vi "Assign Pixel to Wing Sector (Host).vi"(6 "Pixel Intensity In":u8, 7 "Right Wing?":bool, 8 "Sector Parameters":T1, 9 "Pixel Y":u16, 10 "Pixel X":u16) -> (0 "Pixel Y Out":u16, 1 "Pixel Intensity Out":u8, 2 "sector #":u8, 3 "output valid":bool, 4 "Pixel X Out":u16)   [LabVIEW 2013]
uses:
  FPGA/Sector/Accumulate/Sector Parameter Cluster.ctl
  <vilib>/rvi/FXPMathLib/FxpRectToPolar/subVIs/nifxpmath_RectToPolar_SimConfig.ctl
  <vilib>/rvi/FXPMathLib/FxpDiv/subVIs/nifxpmath_Div_SimConfig.ctl
  <vilib>/rvi/FXPMathLib/FxpRectToPolar/simVIs/DllFxpRectToPolarTemp_sub.vi
  <vilib>/rvi/FXPMathLib/FxpDiv/simVIs/DllFxpDivTemp_sub.vi
  <vilib>/rvi/FXPMathLib/FxpSub/XNode/nifxpmath_Sub.xnode
  <vilib>/rvi/FXPMathLib/FxpRectToPolar/XNode/nifxpmath_RectToPolar.xnode
  <vilib>/rvi/FXPMathLib/FxpAdd/XNode/nifxpmath_Add.xnode
  <vilib>/rvi/FXPMathLib/FxpDiv/XNode/nifxpmath_Div.xnode
  <vilib>/rvi/FXPMathLib/sim/FxpSim.dll
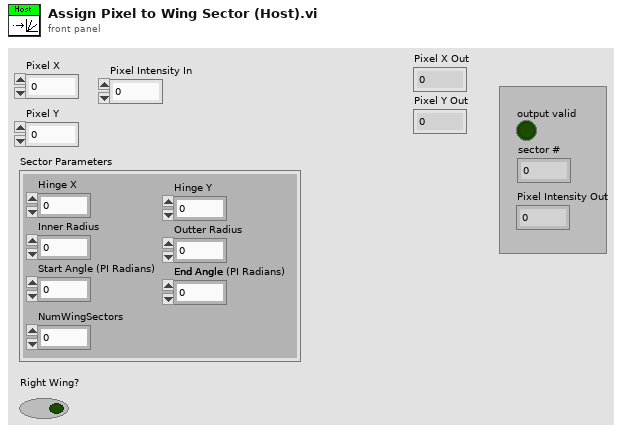
[diagram p1: front panel]
types:
  T1 = typedef "Sector Parameter Cluster.ctl" = cluster{"Start Angle":fxp<+/-,17,2>, "End Angle":fxp<+,17,3>, "Inner Radius":u16, "Outter Radius":u16, "Hinge X":u16, "Hinge Y":u16, "NumWingSectors":u8}
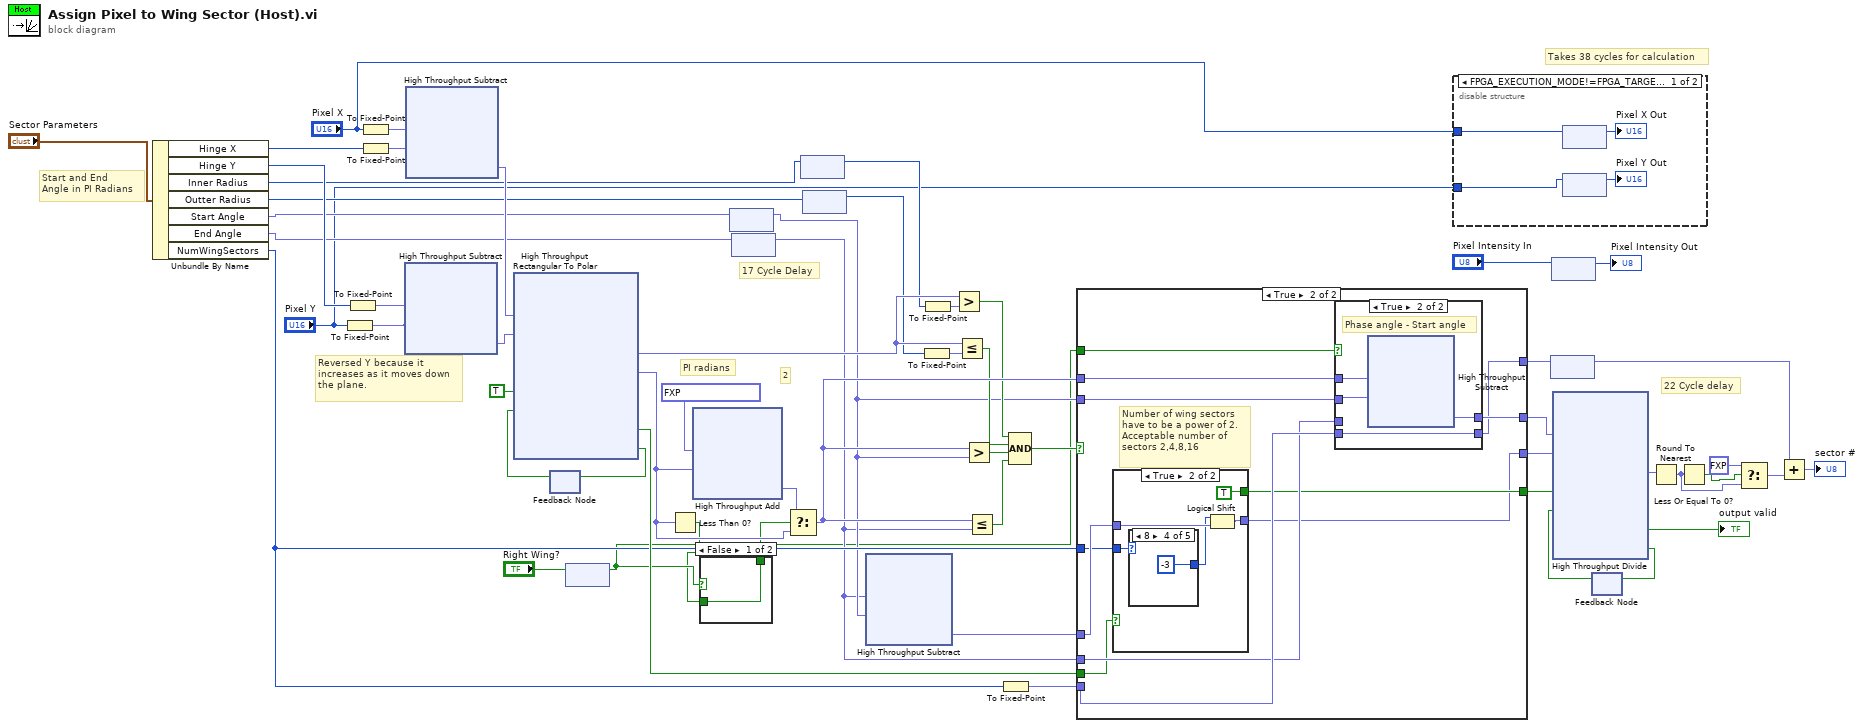
[diagram p0: block diagram]
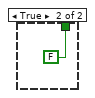
[diagram p2: hidden frame]
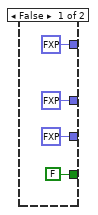
[diagram p4: hidden frame]
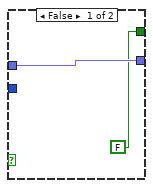
[diagram p5: hidden frame]
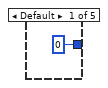
[diagram p6: hidden frame]
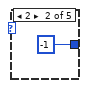
[diagram p7: hidden frame]
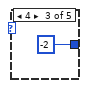
[diagram p8: hidden frame]
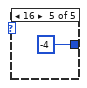
[diagram p9: hidden frame]
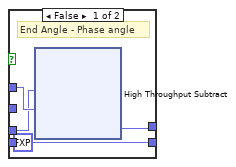
[diagram p10: hidden frame]
diagram:
  # "Takes 38 cycles for calculation"
  # "17 Cycle Delay"
  # "Reversed Y because it\nincreases as it moves down\nthe plane."
  # "PI radians"
  # "22 Cycle delay"
  # "Start and End\nAngle in PI Radians"
  # "2"
  n1 = Unbundle By Name("Sector Parameters") -> ("Hinge X"=w23:u16, "Hinge Y"=w43:u16, "Inner Radius"=w20:u16, "Outter Radius"=w18:u16, "Start Angle"=w16:fxp<+/-,17,2>, "End Angle"=w14:fxp<+,17,3>, "NumWingSectors"=w26:u8)
  n2 = To Fixed-Point(number="Pixel Y") -> (fixed-point=w31:fxp<+,11,11>)  [unwired: 1 in]
  n3 = To Fixed-Point(number=w43) -> (fixed-point=w32:fxp<+,11,11>)  [unwired: 1 in]
  n4 = To Fixed-Point(number="Pixel X") -> (fixed-point=w30:fxp<+,11,11>)  [unwired: 1 in]
  n5 = To Fixed-Point(number=w23) -> (fixed-point=w29:fxp<+,11,11>)  [unwired: 1 in]
  n6 = xnode "High Throughput Subtract"("x"=w32, "y"=w31) -> ("x-y"=w41:fxp<+/-,12,12>)
  n7 = xnode "High Throughput Subtract"("x"=w30, "y"=w29) -> ("x-y"=w40:fxp<+/-,12,12>)
  n8 = feedback #1() -> (w48:bool)  [unwired: 1 in]
  n9 = xnode "High Throughput Rectangular To Polar"("x"=w40, "y"=w41, "input valid"=TRUE, "ready for output (T)"=w48) -> ("magnitude"=w57:fxp<+,12,12>, "phase (pi)"=w54:fxp<+/-,16,2>, "output valid"=w27:bool, "ready for input"=w49:bool)
  n10 = feedback-in #1(w49) -> ()
  n11 = feedback #2() -> (w6:bool)  [unwired: 1 in]
  n12 = feedback-in #2("Right Wing?") -> ()
  n13 = Less Than 0?(x=w54) -> (x < 0?=w5:bool)
  n14 = xnode ("High Throughput Add")("x"=fxp<+/-,16,2> 1.99993896484375 ("y"), "y"=w54) -> ("x+y"=w53:fxp<+/-,17,3>)
  n15 = case shown="False" w6 {
    tunnel: [w59 FALSE ("s")] -> w4
    tunnel: w5 -> [w59 _]
    frame False {
    }
    frame True {
    }
  }
  n16 = feedback #3() -> (w15:fxp<+/-,17,2>)  [unwired: 1 in]
  n17 = feedback-in #3(w16) -> ()
  n18 = feedback #4() -> (w13:fxp<+,17,3>)  [unwired: 1 in]
  n19 = feedback-in #4(w14) -> ()
  n20 = Select(t=w53, s=w4, f=w54) -> (s? t:f=w51:fxp<+/-,17,3>)
  n21 = feedback #5() -> (w19:u16)  [unwired: 1 in]
  n22 = feedback-in #5(w20) -> ()
  n23 = feedback #6() -> (w17:u16)  [unwired: 1 in]
  n24 = feedback-in #6(w18) -> ()
  n25 = xnode ("High Throughput Subtract")("x"=w13, "y"=w15) -> ("x-y"=w28:fxp<+/-,17,6>)
  n26 = To Fixed-Point(number=w17) -> (fixed-point=w56:fxp<+,16,16>)  [unwired: 1 in]
  n27 = To Fixed-Point(number=w19) -> (fixed-point=w58:fxp<+,16,16>)  [unwired: 1 in]
  n28 = Greater?(x=w57, y=w58) -> (0:w47:bool)
  n29 = Less Or Equal?(x=w57, y=w56) -> (x <= y?=w46:bool)
  n30 = Greater?(x=w51, y=w15) -> (0:w45:bool)
  n31 = Less Or Equal?(x=w51, y=w13) -> (x <= y?=w44:bool)
  n32 = To Fixed-Point(number=w26) -> (fixed-point=w42:fxp<+,8,8>)  [unwired: 1 in]
  n33 = Compound Arithmetic op=AND(w47, w46, w45, w44) -> (w55:bool)
  n34 = case shown="True" w55 {
    tunnel: w51 -> [_ w76]
    tunnel: w15 -> [_ w75]
    tunnel: [fxp<+/-,17,6> 0.0 ("x-y") w66] -> w36
    tunnel: w13 -> [_ w73]
    tunnel: w42 -> [_ w74]
    tunnel: [fxp<+/-,19,5> 0.0 ("x-y") w72] -> w37
    tunnel: [FALSE ("output valid") w67] -> w35
    tunnel: [fxp<+,8,8> 0.0 w71] -> w33
    tunnel: w28 -> [_ w70]
    tunnel: w27 -> [_ w69]
    tunnel: w26 -> [_ w68]
    tunnel: w6 -> [_ w65]
    frame False {
    }
    frame True {
      # "Number of wing sectors\nhave to be a power of 2.\nAcceptable number of\nsectors 2,4,8,16"
      n35 = case shown="True" w69 {
        tunnel: w68 -> [_ w83]
        tunnel: w70 -> [w78 w82]
        tunnel: [w78 w80] -> w66
        tunnel: [FALSE ("output valid") TRUE ("output valid")] -> w67
        frame False {
        }
        frame True {
          n36 = case shown="8" w83 {
            tunnel: [i16 0 ("y") i16 -1 ("y") i16 -2 ("y") i16 -3 ("y") i16 -4 ("y")] -> w81
            frame Default {
            }
            frame 2 {
            }
            frame 4 {
            }
            frame 8 {
            }
            frame 16 {
            }
          }
          n37 = Logical Shift(y=w81, x=w82) -> (x << y=w80:fxp<+/-,17,6>)
        }
      }
      n38 = case shown="True" w65 {
        tunnel: w76 -> [w91 w96]
        tunnel: w75 -> [_ w95]
        tunnel: [w92 w94] -> w72
        tunnel: w74 -> [_ w93]
        tunnel: [fxp<+,8,8> 0.0 w93] -> w71
        tunnel: w73 -> [w90 _]
        frame False {
          # "End Angle - Phase angle"
          n39 = xnode "High Throughput Subtract"("x"=w90, "y"=w91) -> ("x-y"=w92:fxp<+/-,19,5>)
        }
        frame True {
          # "Phase angle - Start angle"
          n40 = xnode ("High Throughput Subtract")("x"=w96, "y"=w95) -> ("x-y"=w94:fxp<+/-,19,4>)
        }
      }
    }
  }
  n41 = disable-structure shown="FPGA_EXECUTION_MODE!=FPGA_TARGET" {
    disable-tunnel: "Pixel X" -> [w100 _]
    disable-tunnel: "Pixel Y" -> [w99 _]
    frame condition #0 (active) {
      n42 = feedback #7() -> (→"Pixel X Out":u16)  [unwired: 1 in]
      n43 = feedback-in #7(w100) -> ()
      n44 = feedback #8() -> (→"Pixel Y Out":u16)  [unwired: 1 in]
      n45 = feedback-in #8(w99) -> ()
    }
    frame condition #1 {
    }
  }
  n46 = feedback #9() -> (w10:fxp<+,8,8>)  [unwired: 1 in]
  n47 = feedback-in #9(w33) -> ()
  n48 = feedback #10() -> (→"Pixel Intensity Out":u8)  [unwired: 1 in]
  n49 = feedback-in #10("Pixel Intensity In") -> ()
  n50 = feedback #11() -> (w34:bool)  [unwired: 1 in]
  n51 = xnode "High Throughput Divide"("x"=w37, "y"=w36, "input valid"=w35, "ready for output (T)"=w34) -> ("x/y"=w3:fxp<+/-,20,16>, "output valid"=→"output valid":bool, "ready for input"=w39:bool)
  n52 = feedback-in #11(w39) -> ()
  n53 = Round To Nearest(number=w3) -> (nearest integer value=w1:fxp<+/-,17,17>)
  n54 = Less Or Equal To 0?(x=w1) -> (x <= 0?=w2:bool)
  n55 = Select(t=fxp<+/-,17,17> 1.0, s=w2, f=w1) -> (s? t:f=w12:fxp<+/-,17,17>)
  n56 = Add(x=w10, y=w12) -> (x+y=→"sector #":fxp<+/-,17,17>)
